vi "Post Information.vi"(8 "Error In":errorcluster, 10 "Message":string, 11 "Custom Device Name":string) -> (0 "Error Out":errorcluster)   [LabVIEW 2018]
doc: "Use this VI to post information messages to the System Log."
uses:
  <vilib>/Utility/SystemLogging/NI_SystemLogging.lvlib
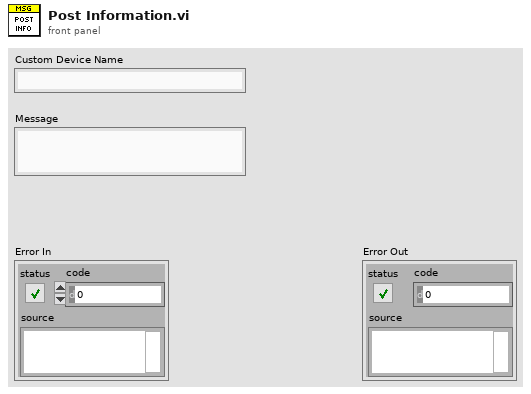
[diagram p1: front panel]
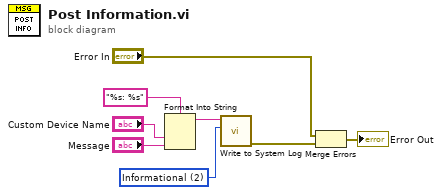
[diagram p0: block diagram]
diagram:
  w3 = 2 items=["Error", "Warning", "Informational"] ("severity")
  n1 = Format Into String(format string="%s: %s", "Custom Device Name", "Message") -> (resulting string=w6:string)  [unwired: 2 in, 1 out]
  n2 = call <vilib>:"Write to System Log.vi"("severity"=w3, "message"=w6) -> ("error out"=w5:errorcluster)  [unwired: 9 in]
  n3 = Merge Errors("Error In", w5) -> (→"Error Out":errorcluster)
